vi "TestWaitLogic.vi"() -> ()   [LabVIEW 2018]
panel:
  out "Call Auto-Hatch":bool
  out "Call Toggle":bool
  in  "Delay":dbl=300.0
  in  "Right Bumper":bool
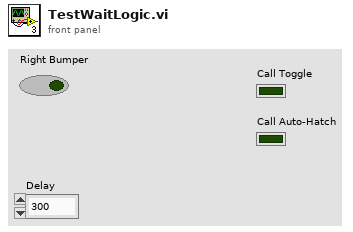
[diagram p1: front panel]
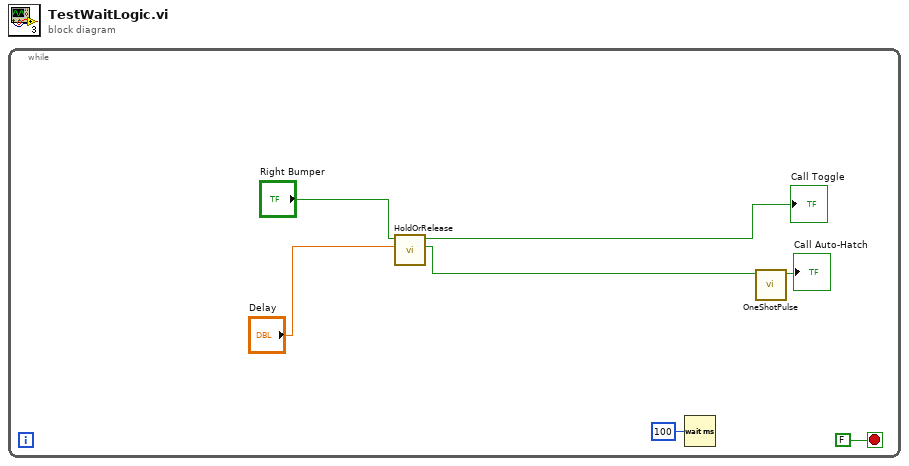
[diagram p0: block diagram]
diagram:
  n1 = while {
    stop <- FALSE stop-if-true
    n2 = call "HoldOrRelease.vi"("Delay"="Delay", "Right Bumper"="Right Bumper") -> ("Call Auto-Hatch"=w2:bool, "Call Toggle"=→"Call Toggle":bool)  [unwired: 8 in]
    n3 = Wait (ms)(milliseconds to wait=u32 100) -> ()  [unwired: 1 out]
    n4 = call "OneShotPulse.vi"("Input"=w2) -> ("Output"=→"Call Auto-Hatch":bool)  [unwired: 10 in]
  }
